vi "WouldCrowdProperty.vi"(8 "error IO":errorcluster, 9 "Wants Write":bool, 10 "WantsRead":bool, 11 "Proposed Folder Refnum in":refnum<vi>) -> (0 "error out":errorcluster, 2 "Would crowd?":bool, 3 "Folder Refnum out":refnum<vi>)   [LabVIEW 2021, in "MemberVICreation.lvlib" / "BaseAccessorScripter.lvclass"]
uses:
  <resource>/Framework/Providers/LVClassLibrary/NewAccessors/BaseAccessorScripter/BaseAccessorScripter.lvclass
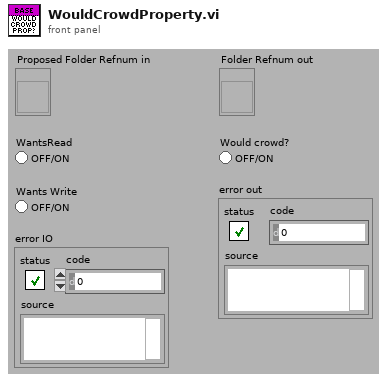
[diagram p1: front panel]
types:
  T1 = enum16{"Invalid Wire Rule", "Required", "Recommended", "Optional", "Dynamic Dispatch"}[]
  T2 = enum16{"Invalid Wire Rule", "Required", "Recommended", "Optional", "Dynamic Dispatch"}
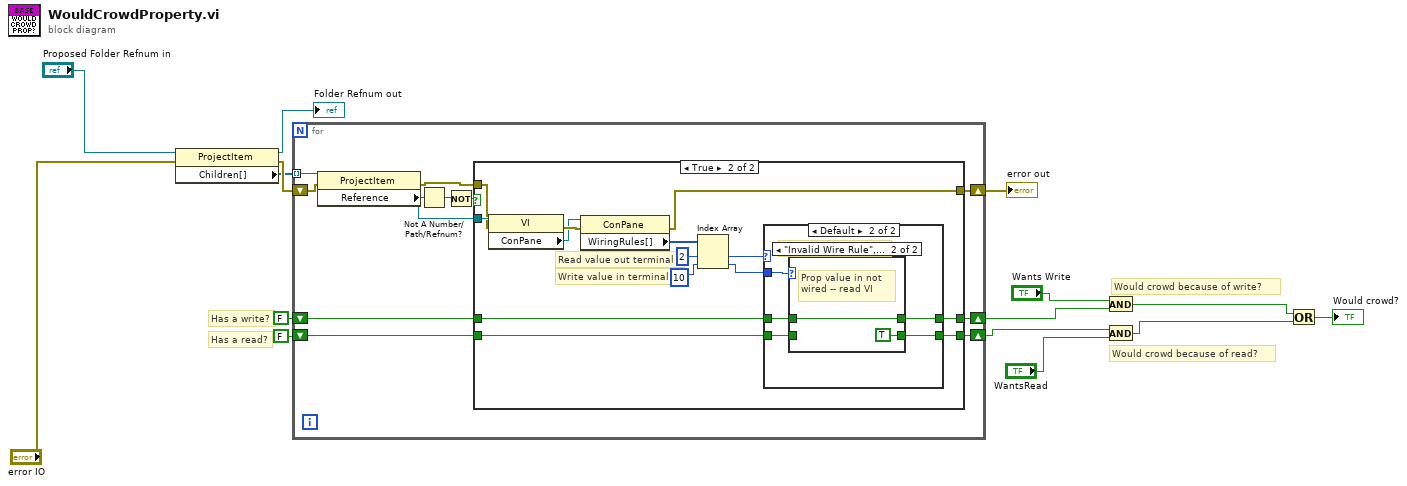
[diagram p0: block diagram]
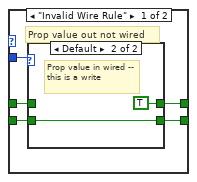
[diagram p3: hidden frame]
diagram:
  # "Would crowd because of read?"
  # "Would crowd because of write?"
  # "Has a read?"
  # "Has a write?"
  n1 = property class="ProjectItem"(reference="Proposed Folder Refnum in", error in="error IO") -> (reference out=→"Folder Refnum out":refnum<vi>, error out=w14:errorcluster, "Children[]"=w2:refnum<vi>[])
  n2 = for {
    tunnel: w2 -> [w26] mode=indexing
    shift-right: [w22] -> w6
    shift-left: FALSE -> [w21]
    shift-right: [w20] -> w7
    shift-left: FALSE -> [w19]
    shift-right: [w16] -> w15
    shift-left: w14 -> [w18]
    n3 = property class="ProjectItem"(reference=w26, error in=w18) -> (error out=w17:errorcluster, "Reference"=w23:refnum<vi>)  [unwired: 1 out]
    n4 = Not A Number/Path/Refnum?(number/path/refnum=w23) -> (NaN/Path/Refnum?=w25:bool)
    n5 = Not(x=w25) -> (.not. x?=w24:bool)
    n6 = case shown="True" w24 {
      tunnel: w23 -> [_ w43]
      tunnel: [w29 w35] -> w22
      tunnel: w21 -> [w29 w34]
      tunnel: [w28 w33] -> w20
      tunnel: w19 -> [w28 w32]
      tunnel: w17 -> [w27 w31]
      tunnel: [w27 w30] -> w16
      frame False {
      }
      frame True {
        # "Write value in terminal"
        # "Read value out terminal"
        n7 = property class="VI"(reference=w43, error in=w31) -> (error out=w42:errorcluster, "ConPane"=w41:refnum<vi>)  [unwired: 1 out]
        n8 = property class="ConPane"(reference=w41, error in=w42) -> (error out=w30:errorcluster, "WiringRules[]"=w40:T1)  [unwired: 1 out]
        n9 = Index Array(array=w40, index #1=2 ("index"), index #2=10 ("index")) -> (element #1=w37:T2, element #2=w36:T2)
        n10 = case shown="Default" w37 {
          tunnel: w36 -> [w48 w57]
          tunnel: [w47 w53] -> w35
          tunnel: w34 -> [w46 w54]
          tunnel: [w44 w56] -> w33
          tunnel: w32 -> [w45 w55]
          frame "Invalid Wire Rule" {
            # "Prop value out not wired"
            n11 = case shown="Default" w48 {
              tunnel: [w50 TRUE] -> w47
              tunnel: w46 -> [w50 _]
              tunnel: w45 -> [w49 w51]
              tunnel: [w49 w51] -> w44
              frame "Invalid Wire Rule" {
                # "Neither wired...bad vi"
              }
              frame Default {
                # "Prop value in wired -- this is a write"
              }
            }
          }
          frame Default {
            # "Prop value out wired"
            n12 = case shown="\"Invalid Wire Rule\", \"Optional\"" w57 {
              tunnel: [w58 TRUE] -> w56
              tunnel: w55 -> [w58 _]
              tunnel: w54 -> [w59 w60]
              tunnel: [w59 w60] -> w53
              frame Default {
                # "Both wired...bad"
              }
              frame "Invalid Wire Rule", "Optional" {
                # "Prop value in not wired -- read VI"
              }
            }
          }
        }
      }
    }
  }
  "error out" <- w15
  n13 = And(x="Wants Write", y=w6) -> (x .and. y?=w10:bool)
  n14 = And(x=w7, y="WantsRead") -> (x .and. y?=w9:bool)
  n15 = Or(x=w10, y=w9) -> (x .or. y?=→"Would crowd?":bool)
